vi "Read ce.vi"(8 "error in (no error)":errorcluster, 11 "CollOffset in":refnum<class "CollOffset.lvclass">) -> (0 "error out":errorcluster, 2 "ce":dbl[unit] min=-0.00048481368110953597 max=0.00048481368110953597, 3 "CollOffset out":refnum<class "CollOffset.lvclass">)   [LabVIEW 2014, in "TCSDataDefinitions.lvlib" / "TCSCommand.lvlib" / "OffsetCommands.lvlib" / "CollOffset.lvclass"]
uses:
  CollOffset.lvclass
  CollOffset.lvclass/CollOffset.ctl
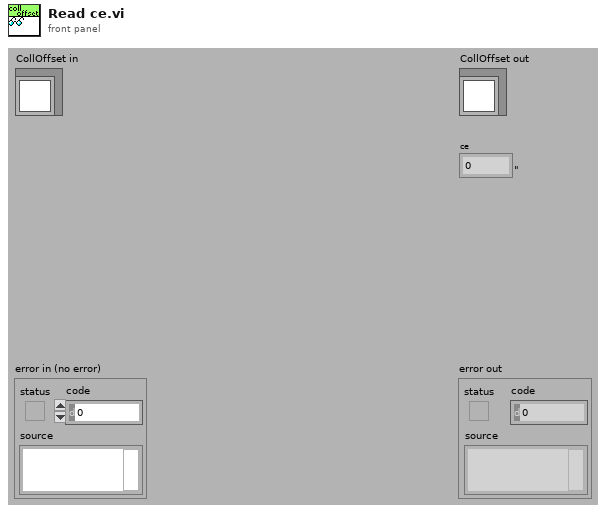
[diagram p1: front panel]
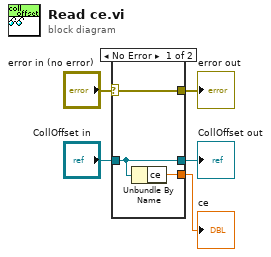
[diagram p0: block diagram]
diagram:
  n1 = case shown="No Error" "error in (no error)" {
    selector: "error in (no error)" -> [w8 w9]
    tunnel: [w8 w9] -> w4
    tunnel: [w7 w10] -> w2
    tunnel: "CollOffset in" -> [w7 w10]
    tunnel: [w6 _] -> w1
    frame No Error {
      n2 = Unbundle By Name(w7) -> ("ce"=w6:dbl[unit])
    }
    frame Error {
    }
  }
  "error out" <- w4
  "CollOffset out" <- w2
  "ce" <- w1
